vi "Remove.vi"(8 "error in (no error)":errorcluster, 11 "Module ID":i32=-1) -> (0 "error out":errorcluster, 2 "found?":bool, 3 "empty":bool)   [LabVIEW 2014, in "GenNet-Client.lvlib" / "Clone Registration.lvlib"]
doc: "Remove the specified cloneable module ID from the registry.\n_____\nBased on Delacor QMH Project Template 3.1.0.34.\n\n<b>Note:</b> This VI was modified by the <b>Validate DQMH Module</b> tool to upgrade it to the DQMH 5.0 approach to destroying cloneable module event references."
uses:
  Clone Registration.lvlib
  Action--enum.ctl
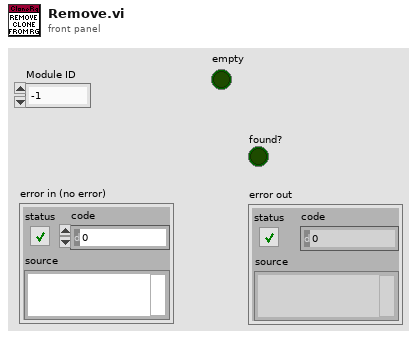
[diagram p1: front panel]
types:
  T1 = typedef "GenNet-Client.lvlib/Clone Registration.lvlib/Action--enum.ctl" = enum16{"Init", "Add Instance", "Remove Instance", "List Instances", "Is First?"}
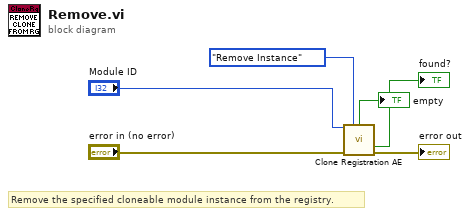
[diagram p0: block diagram]
diagram:
  # "Remove the specified cloneable module instance from the registry."
  n1 = call "Clone Registration AE.vi"("Module ID"="Module ID", "Action"=Action--enum."Remove Instance", "error in (no error)"="error in (no error)") -> ("empty"=→"empty":bool, "Found?"=→"found?":bool, "error out"=→"error out":errorcluster)  [unwired: 4 in, 6 out]
